vi "_Main.vi"   [LabVIEW 2016, in "DashboardComm.lvlib"]
uses:
  DashboardComm.lvlib
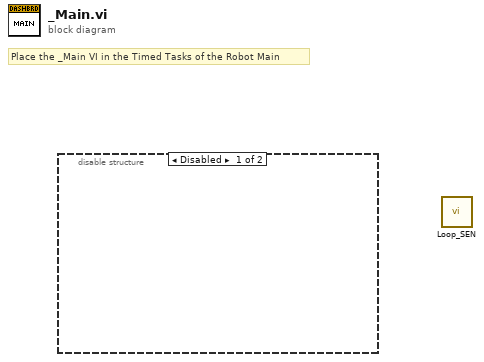
[diagram p0: block diagram]
diagram:
  # "Place the _Main VI in the Timed Tasks of the Robot Main"
  n1 = disable-structure shown="Disabled" {
    frame Disabled {
    }
    frame Enabled {
    }
  }
  n2 = call "Loop_SEN.vi"() -> ()  [unwired: 12 in]
